vi "niRFUtil RFHS Channelizer CreateFineTuneResampler CSG.vi"(2 "Benchmark Task":T5, 5 "fs [Hz]":dbl=1000000000.0 format="%#_6p", 7 "Mode":T1, 9 "Buffer Size (s)":dbl=0.003 format="%#_6p", 11 "error in (no error)":errorcluster) -> (4 "Resampler Ref":refnum<data-value>, 15 "error out":errorcluster)   [LabVIEW 2015, in "niRFUtil.lvlib"]
uses:
  niRFUtil.lvlib
  Utilities/Benchmark/niRFUtil RFHS Benchmark Task.ctl
  Utilities/niRFUtil RFHS Util User Filter Specification.ctl
  Includes/niRFUtil RFHS Channelizer ChannelSpecificationBase.ctl
  Includes/niRFUtil RFHS Channelizer ChannelFlags.ctl
  Includes/niRFUtil RFHS Channelizer ChannelizerBufferingMode.ctl
  Includes/niRFUtil RFHS Channelizer ResamplerInfo CSG.ctl
  Includes/niRFUtil RFHS Channelizer FilterRef.ctl
  Utilities/Data FIFO/niRFUtil RFHS FIFO Reference.ctl
  Utilities/Data FIFO/niRFUtil RFHS FIFO.ctl
  Includes/niRFUtil RFHS Channelizer ChannelizerFlags.ctl
  Includes/niRFUtil RFHS Channelizer FilterSpecification.ctl
panel:
  in  "Inital Phase":dbl
  in  "Channel Spec Base":T2={"fc"=0.0, "fs"=1.0, "passBW"=0.8, "stopBW"=0.0012, "Rejection (dB)"=85.0, "Flags"=0, "Reserved"=0} {"Flags" items=["None"=0, "Force Fractional"=1, "Use Multistage"=2, "Use Pretrigger Data "=256, "Frequency Shift Only"=4]; "fs" format="%#_8p"; "fc" format="%#_6p"; "stopBW" format="%#_6p"; "passBW" format="%#_6p"}
  in  "User Filter Spec":T4
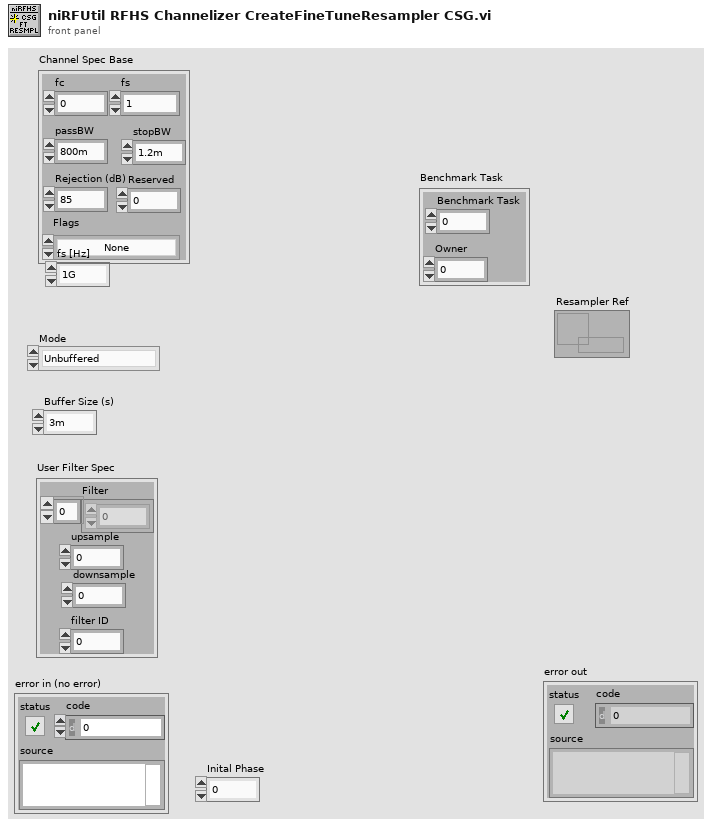
[diagram p1: front panel]
types:
  T1 = typedef "niRFUtil.lvlib/niRFUtil RFHS Channelizer ChannelizerBufferingMode.ctl" = enum32{"Unbuffered", "Finite", "Continuous"}
  T2 = typedef "niRFUtil.lvlib/niRFUtil RFHS Channelizer ChannelSpecificationBase.ctl" = cluster{"fc":dbl, "fs":dbl, "passBW":dbl, "stopBW":dbl, "Rejection (dB)":dbl, "Flags":T3, "Reserved":i32}
  T3 = typedef "niRFUtil.lvlib/niRFUtil RFHS Channelizer ChannelFlags.ctl" = u32
  T4 = typedef "niRFUtil.lvlib/niRFUtil RFHS Util User Filter Specification.ctl" = cluster{"Filter":dbl[], "upsample":i32, "downsample":i32, "filter ID":i32}
  T5 = typedef "niRFUtil.lvlib/niRFUtil RFHS Benchmark Task.ctl" = cluster{"Benchmark Task":u64, "Owner":u32}
  T6 = enum16{"Reserved", "Rational", "Fine Tune", "Fractional"}
  T7 = typedef "niRFUtil.lvlib/niRFUtil RFHS Channelizer FilterSpecification.ctl" = cluster{"Type":enum32{"Reserved", "Rational", "Fine Tune", "Fractional", "Rational (user)", "Reserved 2", "Fractional (user)", "FFT Resampler"}, "Reserved":i32, "Spec":T2}
  T8 = typedef "niRFUtil.lvlib/niRFUtil RFHS Channelizer ResamplerInfo CSG.ctl" = cluster{"Filter LVRef":T9, "Mode":T1, "History":csg[], "Buffer":csg[], "FIFO":T10, "BufferW":u32, "BufferR":u32, "Phase":dbl, "Flags":T12, "Reset Cnt":i64}
  T9 = typedef "niRFUtil.lvlib/niRFUtil RFHS Channelizer FilterRef.ctl" = cluster{"Ref":u64, "GUID":u64, "Upsample":i32, "Downsample":i32, "Size":i32, "Num Taps":i32}
  T10 = typedef "niRFUtil.lvlib/niRFUtil RFHS FIFO Reference.ctl" = cluster{"Read Lock":refnum<data-value>, "Info":T11, "Write Lock":refnum<data-value>}
  T11 = typedef "niRFUtil.lvlib/niRFUtil RFHS FIFO.ctl" = cluster{"ID":u64, "Length":u32}
  T12 = typedef "niRFUtil.lvlib/niRFUtil RFHS Channelizer ChannelizerFlags.ctl" = u32
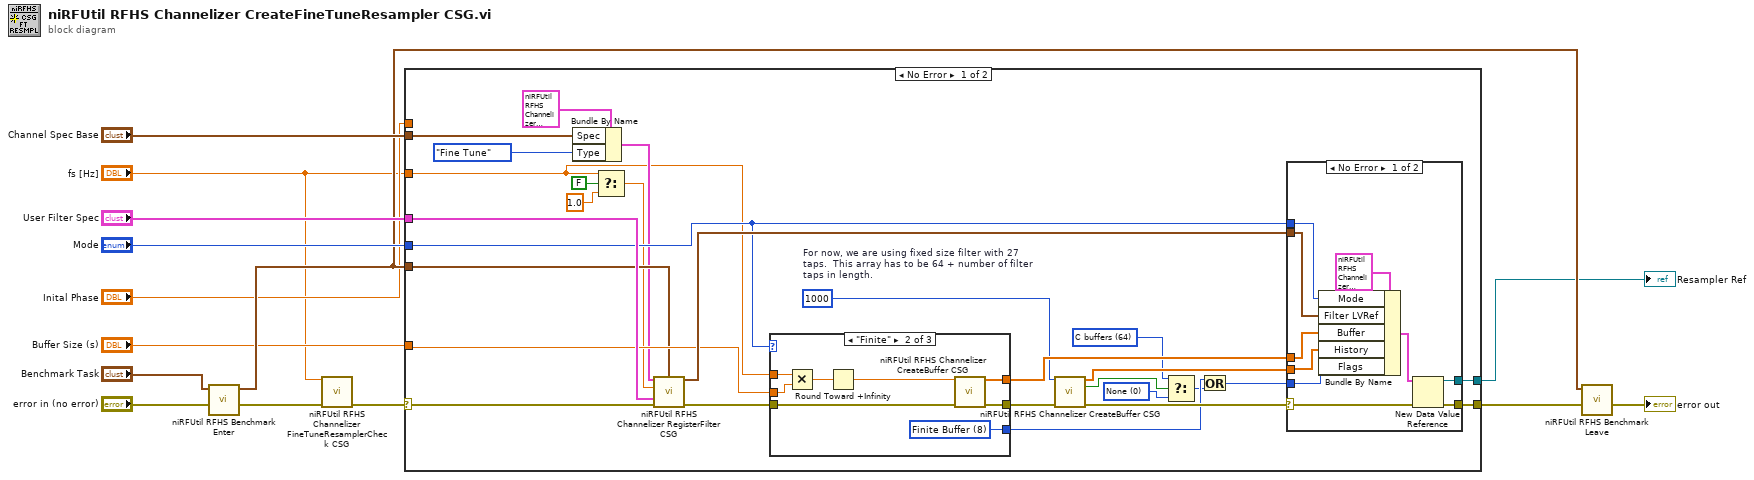
[diagram p0: block diagram]
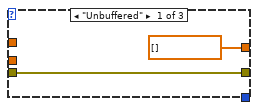
[diagram p3: hidden frame]
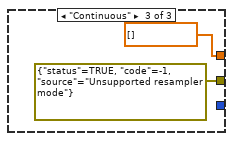
[diagram p4: hidden frame]
diagram:
  n1 = call "niRFUtil RFHS Benchmark Enter.vi"("error in (no error)"="error in (no error)", "Benchmark Task (Parent)"="Benchmark Task") -> ("error out"=w3:errorcluster, "Benchmark Task (Self)"=w7:T5)  [unwired: 8 in]
  n2 = call "niRFUtil RFHS Channelizer FineTuneResamplerCheck CSG.vi"("fs [Hz]"="fs [Hz]", "error in (no error)"=w3) -> ("error out"=w2:errorcluster)  [unwired: 13 in]
  n3 = case shown="No Error" w2 {
    selector: w2 -> [w42 w66]
    tunnel: [w25 w66] -> w13
    tunnel: "Channel Spec Base" -> [w30 _]
    tunnel: "fs [Hz]" -> [w26 _]
    tunnel: "User Filter Spec" -> [w41 _]
    tunnel: "Mode" -> [w38 _]
    tunnel: w7 -> [w34 _]
    tunnel: [w40 _] -> w4
    tunnel: "Buffer Size (s)" -> [w35 _]
    tunnel: "Inital Phase" -> [_ _]
    frame No Error {
      w17 = T12 0 items=["None"=0, "Skip Stage 1"=1, "FFT Stage"=2, "Frequency Shift"=4, "Finite Buffer"=8, "Reset"=16, "Input Len Estimate"=32, "C buffers"=64, "Input From Ref"=128] ("Flags")
      w18 = T12 64 items=["None"=0, "Skip Stage 1"=1, "FFT Stage"=2, "Frequency Shift"=4, "Finite Buffer"=8, "Reset"=16, "Input Len Estimate"=32, "C buffers"=64, "Input From Ref"=128] ("Flags")
      w22 = 1000  # For now, we are using fixed size filter with 27 taps.  This array has to be 64 + number of filter taps in length.
      n4 = Bundle By Name(cluster=T7 {"Type"=enum."Reserved", "Reserved"=0, "Spec"={"fc"=0.0, "fs"=0.0, "passBW"=0.0, "stopBW"=0.0, "Rejection (dB)"=0.0, "Flags"=0, "Reserved"=0}} ("Filter Spec"), "Spec"=w30, "Type"=T6."Fine Tune") -> (w28:T7)
      n5 = Select(t=w26, s=FALSE, f=1.0 ("t")) -> (s? t:f=w32:dbl)
      n6 = call "niRFUtil RFHS Channelizer RegisterFilter CSG.vi"("Filter Spec"=w28, "Benchmark Task"=w34, "fs"=w32, "User Filter Spec"=w41, "error in (no error)"=w42) -> ("Filter LVRef"=w39:T9, "error out"=w36:errorcluster)  [unwired: 9 in]
      n7 = case shown="\"Finite\"" w38 {
        tunnel: [csg[] [] w56 csg[] []] -> w37
        tunnel: w36 -> [w54 w58 _]
        tunnel: [w54 w57 errorcluster {"status"=TRUE, "code"=-1, "source"="Unsupported resampler mode"} ("error out")] -> w24
        tunnel: w35 -> [_ w62 _]
        tunnel: w26 -> [_ w63 _]
        tunnel: [_ w60 _] -> w20
        frame "Unbuffered" {
        }
        frame "Finite" {
          w60 = T12 8 items=["None"=0, "Skip Stage 1"=1, "FFT Stage"=2, "Frequency Shift"=4, "Finite Buffer"=8, "Reset"=16, "Input Len Estimate"=32] ("Flags")
          n8 = Multiply(x=w63, y=w62) -> (x*y=w61:dbl)
          n9 = Round Toward +Infinity(x=w61) -> (ceil(x): smallest int >= x=w59:dbl)
          n10 = call "niRFUtil RFHS Channelizer CreateBuffer CSG.vi"("Size"=w59, "error in (no error)"=w58) -> ("Buffer"=w56:csg[], "error out"=w57:errorcluster)  [unwired: 11 in, 1 out]
        }
        frame "Continuous" {
        }
      }
      n11 = call "niRFUtil RFHS Channelizer CreateBuffer CSG.vi"("Size"=w22, "error in (no error)"=w24) -> ("Buffer"=w21:csg[], "Embedded?"=w19:bool, "error out"=w23:errorcluster)  [unwired: 11 in]
      n12 = Select(t=w18, s=w19, f=w17) -> (s? t:f=w16:T12)
      n13 = Or(x=w20, y=w16) -> (x .or. y?=w15:T12)
      n14 = case shown="No Error" w23 {
        selector: w23 -> [w48 w53]
        tunnel: [w51 _] -> w40
        tunnel: w39 -> [w50 _]
        tunnel: w21 -> [w43 _]
        tunnel: w38 -> [w44 _]
        tunnel: w37 -> [w46 _]
        tunnel: w15 -> [w49 _]
        tunnel: [w47 w53] -> w25
        frame No Error {
          n15 = Bundle By Name(cluster=T8 {"Filter LVRef"={"Ref"=0, "GUID"=0, "Upsample"=0, "Downsample"=0, "Size"=0, "Num Taps"=0}, "Mode"=enum."Continuous", "History"=[], "Buffer"=[], "FIFO"={"Read Lock"=refnum, "Info"={"ID"=0, "Length"=0}, "Write Lock"=refnum}, "BufferW"=0, "BufferR"=0, "Phase"=0.0, "Flags"=0, "Reset Cnt"=0} ("Info"), "Mode"=w44, "Filter LVRef"=w50, "Buffer"=w46, "History"=w43, "Flags"=w49) -> (w52:T8)
          n16 = New Data Value Reference(data value=w52, error in=w48) -> (data value reference=w51:refnum<data-value>, error out=w47:errorcluster)
        }
        frame Error {
        }
      }
    }
    frame Error {
    }
  }
  "Resampler Ref" <- w4
  n17 = call "niRFUtil RFHS Benchmark Leave.vi"("error in (no error)"=w13, "Benchmark Task Self"=w7) -> ("error out"=→"error out":errorcluster)  [unwired: 8 in, 1 out]
